vi "Fuel PID Control.vi"(7 "Pressure Controls":T1 {"output range"."output low" format="%.2f"; "output range"."output high" format="%.2f"; "PID gains"."derivative time (Td, min)" format="%.6f"; "PID gains"."integral time (Ti, min)" format="%.5f"; "PID gains"."proportional gain (Kc)" format="%.3f"; "Phi" scale=0.0..1.5; "Des P drop" scale=0.0..6.0}, 8 "Error In":errorcluster) -> (0 "Error Out":errorcluster, 5 "Pressure Indicators":T3 {"Measured Pressure (psi abs)" scale=0.0..6.0})   [LabVIEW 2013]
doc: "This sub-VI reads measured pressures in the fuel system and lab, as well as input control parameters, and\ndetermines the controller effort (voltage) to send to air flow and fuel valves. In short, this sub-VI controls\nthe fuel and air flow to match user inputs."
uses:
  Controls/pressure_indicator_cluster.ctl
  Controls/pressure_control_cluster.ctl
  Controls/run_mode_enum.ctl
  <vilib>/DAQmx/read.llb/DAQmx Read (Analog DBL 1Chan 1Samp).vi
  <vilib>/DAQmx/write.llb/DAQmx Write (Analog DBL 1Chan 1Samp).vi
  <vilib>/addons/control/pid/pid.llb/PID (DBL).vi
  <vilib>/DAQmx/miscellaneous.llb/DAQmx Fill In Error Info.vi
  <vilib>/addons/control/pid/NI_PID_pid.lvlib
  <vilib>/ptbypt/NI_PtbyPt.lvlib
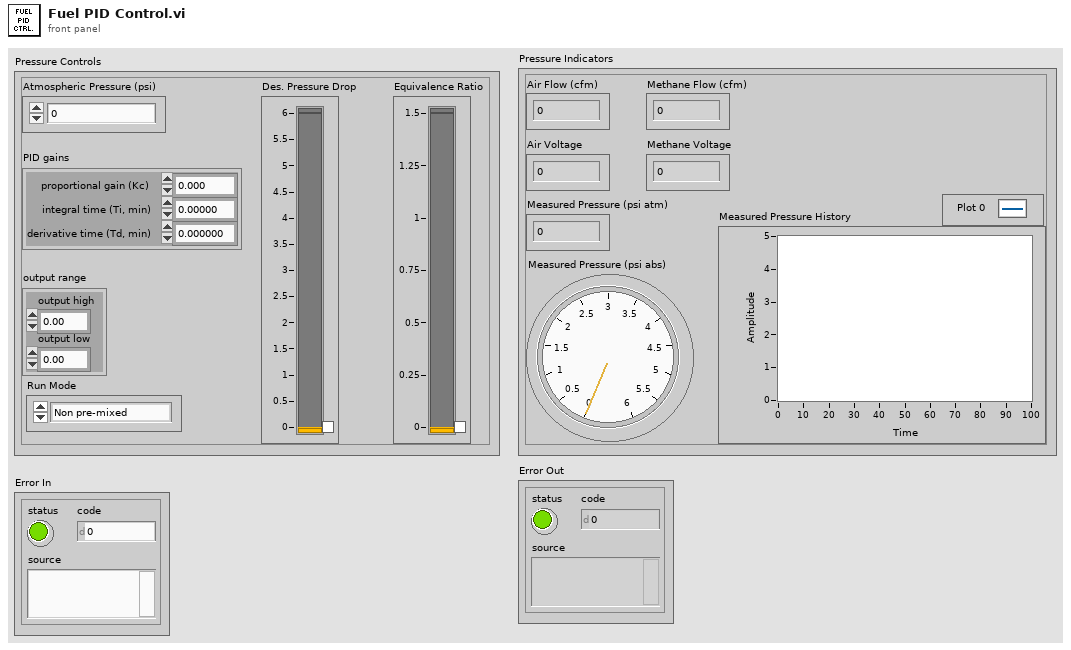
[diagram p1: front panel]
types:
  T1 = typedef "pressure_control_cluster.ctl" = cluster{"Atm Press":dbl, "Des P drop":dbl, "Phi":dbl, "PID gains":cluster{"proportional gain (Kc)":dbl, "integral time (Ti, min)":dbl, "derivative time (Td, min)":dbl}, "output range":cluster{"output high":dbl, "output low":dbl}, "Run Mode":T2}
  T2 = typedef "run_mode_enum.ctl" = enum16{"Non pre-mixed", "Pre-mixed"}
  T3 = typedef "pressure_indicator_cluster.ctl" = cluster{"Air Flow (cfm)":dbl, "Methane Flow (cfm)":dbl, "Air Voltage":dbl, "Methane Voltage":dbl, "Measured Pressure (psi atm)":dbl, "Measured Pressure (psi abs) ":dbl, "Measured Pressure History":dbl}
  T4 = cluster{"proportional gain (Kc)":dbl, "integral time (Ti, min)":dbl, "derivative time (Td, min)":dbl}
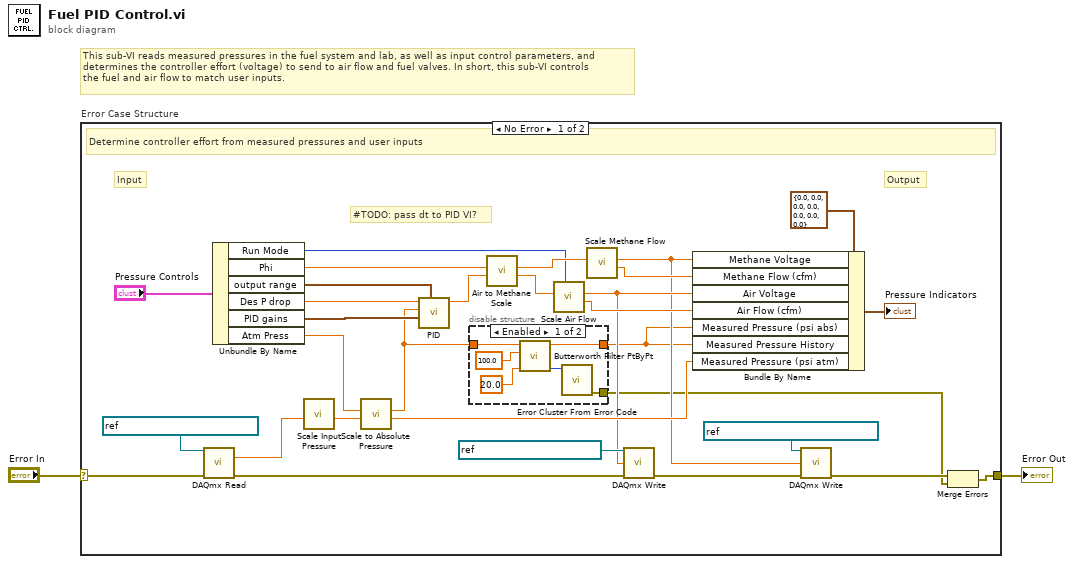
[diagram p0: block diagram]
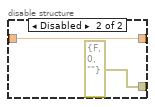
[diagram p2: hidden frame]
diagram:
  # "This sub-VI reads measured pressures in the fuel system and lab, as well as input control parameters, and\ndetermines the controller effort (voltage) to send to air flow and fuel valves. In short, this sub-VI controls\nthe fuel and air flow to match user inputs."
  n1 = case "Error Case Structure" shown="No Error" "Error In" {
    selector: "Error In" -> [w29 w41]
    tunnel: [w4 w41] -> w1
    frame No Error {
      # "#TODO: pass dt to PID VI?"
      # "Output"
      # "Input"
      # "Determine controller effort from measured pressures and user inputs"
      n2 = call-poly <vilib>:"DAQmx Read.vi"("task/channels in"=refnum<k21> "PressureVoltageIn_S3AI8", "error in"=w29) -> ("data"=w17:dbl, "error out"=w21:errorcluster)  [unwired: 11 in, 1 out]
      n3 = Unbundle By Name("Pressure Controls") -> ("Run Mode"=w3:T2, "Phi"=w16:dbl, "output range"=w27:cluster{"output high":dbl, "output low":dbl}, "Des P drop"=w22:dbl, "PID gains"=w28:T4, "Atm Press"=w20:dbl)
      n4 = call "Scale Input Pressure.vi"("Pressure (V)"=w17) -> ("Pressure (psi atm)"=w19:dbl)  [unwired: 10 in]
      n5 = call "Scale to Absolute Pressure.vi"("Pressure (psi atm)"=w19, "Atm Press"=w20) -> ("Pressure out (psi atm)"=w18:dbl, "Pressure (psi abs)"=w8:dbl)  [unwired: 8 in]
      n6 = call-poly <vilib>:"PID.vi"("output range"=w27, "PID gains"=w28, "process variable"=w8, "setpoint"=w22) -> ("output"=w14:dbl)  [unwired: 6 in, 1 out]
      n7 = disable-structure shown="Enabled" {
        disable-tunnel: w8 -> [w38 w40]
        disable-tunnel: [w37 w40] -> w7
        disable-tunnel: [w34 errorcluster {"status"=FALSE, "code"=0, "source"=""} ("error out")] -> w5
        frame Enabled {
          n8 = call <vilib>:"Butterworth Filter PtByPt.vi"("low cutoff freq: fl"=20.0, "sampling freq: fs"=100.0, "x"=w38) -> ("error"=w35:i32, "Filtered x"=w37:dbl)  [unwired: 6 in]
          n9 = call <vilib>:"Error Cluster From Error Code.vi"("error code (0)"=w35) -> ("error out"=w34:errorcluster)  [unwired: 8 in]
        }
        frame Disabled {
        }
      }
      n10 = call "Air to Methane Scale.vi"("Air Flow (cfm)"=w14, "Phi"=w16) -> ("Air Flow (cfm) out"=w13:dbl, "Methane Flow (cfm)"=w15:dbl)  [unwired: 8 in]
      n11 = call "Scale Air Flow.vi"("Run Mode"=w3, "Air Flow (cfm)"=w13) -> ("Air Flow (cfm) out"=w11:dbl, "Air Voltage out"=w10:dbl)  [unwired: 8 in]
      n12 = call "Scale Methane Flow.vi"("Methane flow (cfm)"=w15) -> ("Methan Flow (cfm) out"=w12:dbl, "Methane Voltage out"=w9:dbl)  [unwired: 9 in]
      n13 = call-poly <vilib>:"DAQmx Write.vi"("task/channels in"=refnum<k21> "AirVoltageOut_S3AO0", "data"=w10, "error in"=w21) -> ("error out"=w25:errorcluster)  [unwired: 10 in, 2 out]
      n14 = Bundle By Name(cluster=T3 {"Air Flow (cfm)"=0.0, "Methane Flow (cfm)"=0.0, "Air Voltage"=0.0, "Methane Voltage"=0.0, "Measured Pressure (psi atm)"=0.0, "Measured Pressure (psi abs) "=0.0, "Measured Pressure History"=0.0} ("Pressure Indicators 2"), "Methane Voltage"=w9, "Methane Flow (cfm)"=w12, "Air Voltage"=w10, "Air Flow (cfm)"=w11, "Measured Pressure (psi abs)"=w7, "Measured Pressure History"=w7, "Measured Pressure (psi atm)"=w18) -> (→"Pressure Indicators":T3)
      n15 = call-poly <vilib>:"DAQmx Write.vi"("task/channels in"=refnum<k21> "MethaneVoltageOut_S3AO1", "data"=w9, "error in"=w25) -> ("error out"=w6:errorcluster)  [unwired: 10 in, 2 out]
      n16 = Merge Errors(w6, w5) -> (w4:errorcluster)
    }
    frame Error {
      # "Pass through and exit"
    }
  }
  "Error Out" <- w1
